vi "Multichannel Recording0.9EP.vi"() -> ()   [LabVIEW 2014]
uses:
  Consumer Data_ Consumer Event Com.ctl
  Data Producer States.ctl
  Enum State Typedef.ctl
  <vilib>/_DAQmxBase/Internals/DAQmxBase Read (Analog 2D DBL NChan NSamp).vi
  <vilib>/_DAQmxBase/Internals/DAQmxBase Create Channel (AI-Voltage-Basic).vi
  <vilib>/_DAQmxBase/Internals/DAQmxBase Timing (Sample Clock).vi
panel:
  out "Recording Progress (% )":dbl(slide) scale=0.0..1.0
  in  "Display Size":T1(ring)
  out "Data Producer State":T2=enum."Default"
  out "Data Consumer State":T3=enum."Default"
  in  "Open Button":bool
  in  "Tab Control":T4(tab)
  in  "Amplifier Channel 0":T5 {"Amplifier Model" items=["Select a Model", "AM 1700", "BMA 200"]}
  out "Channel 0 Graph":waveform(dbl)(graph)
  in  "User Data Channel 0":T6
  in  "Use Channel 0":bool caption="In Use?"
  out "Channel 1 Graph":waveform(dbl)(graph)
  in  "User Data Channel 1":T6
  in  "Amplifier Channel 1":T5 {"Amplifier Model" items=["Select a Model", "AM 1700", "BMA 200"]}
  in  "Use Channel 1":bool caption="In Use?"
  out "Channel 2 Graph":waveform(dbl)(graph)
  in  "User Data Channel 2":T6
  in  "Amplifier Channel 2":T5 {"Amplifier Model" items=["Select a Model", "AM 1700", "BMA 200"]}
  in  "Use Channel 2":bool caption="In Use?"
  out "Channel 3 Graph":waveform(dbl)(graph)
  in  "User Data Channel 3":T6
  in  "Amplifier Channel 3":T5 {"Amplifier Model" items=["Select a Model", "AM 1700", "BMA 200"]}
  in  "Use Channel 3":bool caption="In Use?"
  out "Overview Graph":waveform(dbl)[](graph)
  in  "Stop Preview":bool
  in  "OK Button":bool
  in  "Clear Display":bool
  in  "Preview Button":bool
  in  "Recording Time (s)":dbl
  in  "Sample Rate":i64=1000
  in  "Stop Button":bool
  out "Start Time hr/min":string
  out "Date mm/dd/yy":string
  in  "Exit Button":bool
  in  "Record Button":bool
  # "MSU EFISH Lab Multi-Channel Electronic Pulse Recorder v0.9E (Beta 6)"
  # "Setup"
  # "Must set sample rate before you press start"
  # "Preview"
  # "Recording"
  # "Blue for On\nOrange for Off"
  # "DC"
  # "AC"
  # "Blue for AC and Orange for DC"
  # "Blue for On\nOrange for Off"
  # "DC"
  # "AC"
  # "Blue for AC and Orange for DC"
  # "Blue for On\nOrange for Off"
  # "DC"
  # "AC"
  # "Blue for AC and Orange for DC"
  # "Blue for On\nOrange for Off"
  # "DC"
  # "AC"
  # "Blue for AC and Orange for DC"
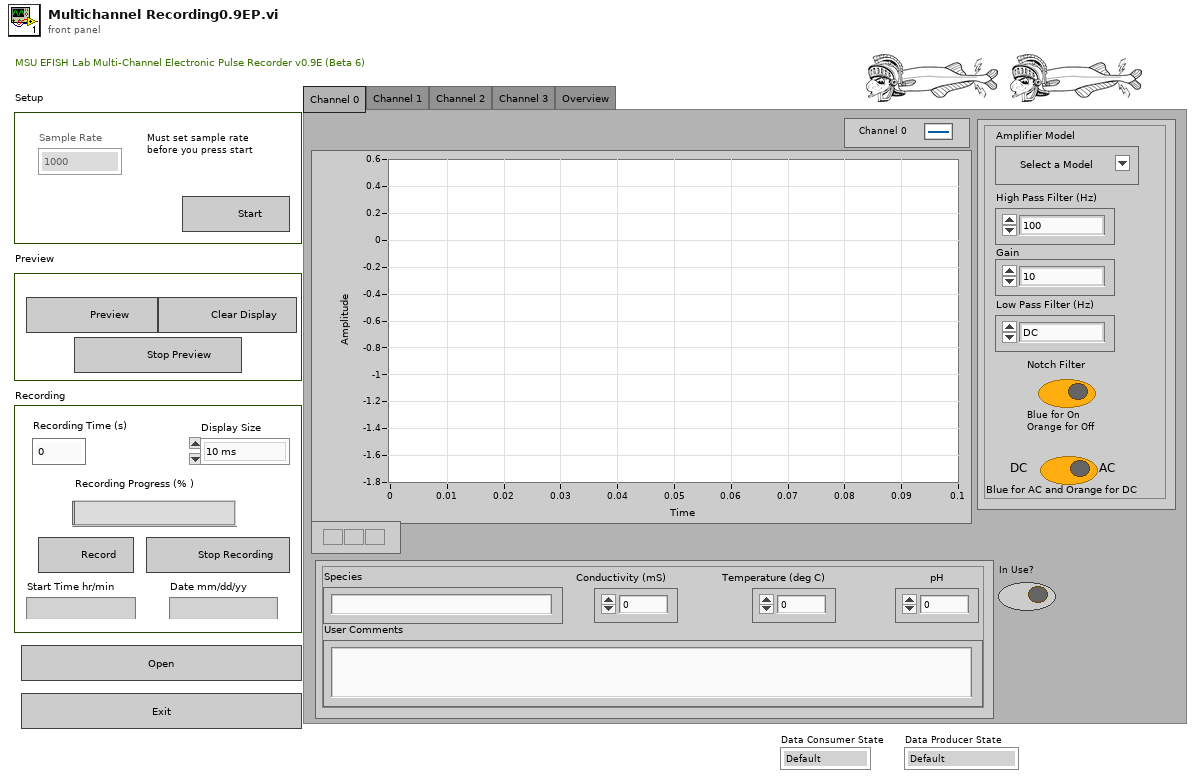
[diagram p1: front panel]
types:
  T1 = enum16{"10 ms", "100 ms", "1 Second", "10 sec", "30 sec"}
  T2 = typedef "Data Producer States.ctl" = enum16{"Read Data", "Set Sample Clock", "Default", "Exit", "Preview"}
  T3 = typedef "Consumer Data_ Consumer Event Com.ctl" = enum16{"Recording", "Create File", "Clear Memory", "Default", "End File", "Exit", "Set Sample Clock", "Preview"}
  T4 = enum32{"Channel 0", "Channel 1", "Channel 2", "Channel 3", "Overview"}
  T5 = cluster{"Low Pass Filter (Hz)":enum16{"DC", "0.1", "1", "3", "10", "30", "100", "300"}, "Gain ":enum16{"10", "20", "50", "100", "200", "500", "1000", "2k", "5k", "10k", "20k", "50k"}, "High Pass Filter (Hz)":enum16{"100", "500", "1000", "3000", "5000", "10,000", "20,000", "30,000", "50,000"}, "Notch Filter":bool, "Amplifier Model":u16, "AC/DC Switch":bool}
  T6 = cluster{"pH":dbl, "Conductivity (mS)":dbl, "Temperature (deg C)":dbl, "User Comments":string, "Species":string}
  T7 = enum8{"Enabled", "Disabled", "Disabled and Grayed Out"}
  T8 = cluster{"Overview Graph":refnum<vi>, "Channel 3 Graph":refnum<vi>, "Channel 2 Graph":refnum<vi>, "Channel 1 Graph":refnum<vi>, "Channel 0 Graph":refnum<vi>}
  T9 = typedef "Enum State Typedef.ctl" = enum16{"Default", "Open FIle", "Beginning State", "Set the Sample Clock", "Prepreview Handling", "Clear Display", "Preview Data", "Stop", "Exit", "Record", "Create File"}
  T10 = enum16{"Recording", "Create File", "Clear Memory", "Default"}
  T11 = cluster{"Refnum out":refnum<k34>, "Refnum out":refnum<k34>, "Refnum out":refnum<k34>, "Refnum out":refnum<k34>}
  T12 = cluster{"Use Channel 0":bool, "Use Channel 1":bool, "Use Channel 2":bool, "Use Channel 3":bool}
  T13 = cluster{"Waveform":waveform(dbl), "Waveform":waveform(dbl), "Waveform":waveform(dbl), "Waveform":waveform(dbl), waveform(dbl)[]}
  T14 = cluster{"tdms file out":refnum<k34>, "tdms file out":refnum<k34>, "tdms file out":refnum<k34>, "tdms file out":refnum<k34>}
  T15 = cluster{"User Data Channel 0":cluster{"pH":dbl, "Conductivity (mS)":dbl, "Temperature (deg C)":dbl, "User Comments":string, "Species":string}, "Amplifier Channel 0":cluster{"Low Pass Filter (Hz)":enum16{"DC", "0.1", "1", "3", "10", "30", "100", "300"}, "Gain ":enum16{"10", "20", "50", "100", "200", "500", "1000", "2k", "5k", "10k", "20k", "50k"}, "High Pass Filter (Hz)":enum16{"100", "500", "1000", "3000", "5000", "10,000", "20,000", "30,000", "50,000"}, "Notch Filter":bool, "Amplifier Model":u16, "AC/DC Switch":bool}, "User Data Channel 1":cluster{"pH":dbl, "Conductivity (mS)":dbl, "Temperature (deg C)":dbl, "User Comments":string, "Species":string}, "Amplifier Channel 1":cluster{"Low Pass Filter (Hz)":enum16{"DC", "0.1", "1", "3", "10", "30", "100", "300"}, "Gain ":enum16{"10", "20", "50", "100", "200", "500", "1000", "2k", "5k", "10k", "20k", "50k"}, "High Pass Filter (Hz)":enum16{"100", "500", "1000", "3000", "5000", "10,000", "20,000", "30,000", "50,000"}, "Notch Filter":bool, "Amplifier Model":u16, "AC/DC Switch":bool}, "User Data Channel 2":cluster{"pH":dbl, "Conductivity (mS)":dbl, "Temperature (deg C)":dbl, "User Comments":string, "Species":string}, "Amplifier Channel 2":cluster{"Low Pass Filter (Hz)":enum16{"DC", "0.1", "1", "3", "10", "30", "100", "300"}, "Gain ":enum16{"10", "20", "50", "100", "200", "500", "1000", "2k", "5k", "10k", "20k", "50k"}, "High Pass Filter (Hz)":enum16{"100", "500", "1000", "3000", "5000", "10,000", "20,000", "30,000", "50,000"}, "Notch Filter":bool, "Amplifier Model":u16, "AC/DC Switch":bool}, "User Data Channel 3":cluster{"pH":dbl, "Conductivity (mS)":dbl, "Temperature (deg C)":dbl, "User Comments":string, "Species":string}, "Amplifier Channel 3":cluster{"Low Pass Filter (Hz)":enum16{"DC", "0.1", "1", "3", "10", "30", "100", "300"}, "Gain ":enum16{"10", "20", "50", "100", "200", "500", "1000", "2k", "5k", "10k", "20k", "50k"}, "High Pass Filter (Hz)":enum16{"100", "500", "1000", "3000", "5000", "10,000", "20,000", "30,000", "50,000"}, "Notch Filter":bool, "Amplifier Model":u16, "AC/DC Switch":bool}}
  T16 = enum16{"Read Data", "Set Sample Clock", "Default", "Exit"}
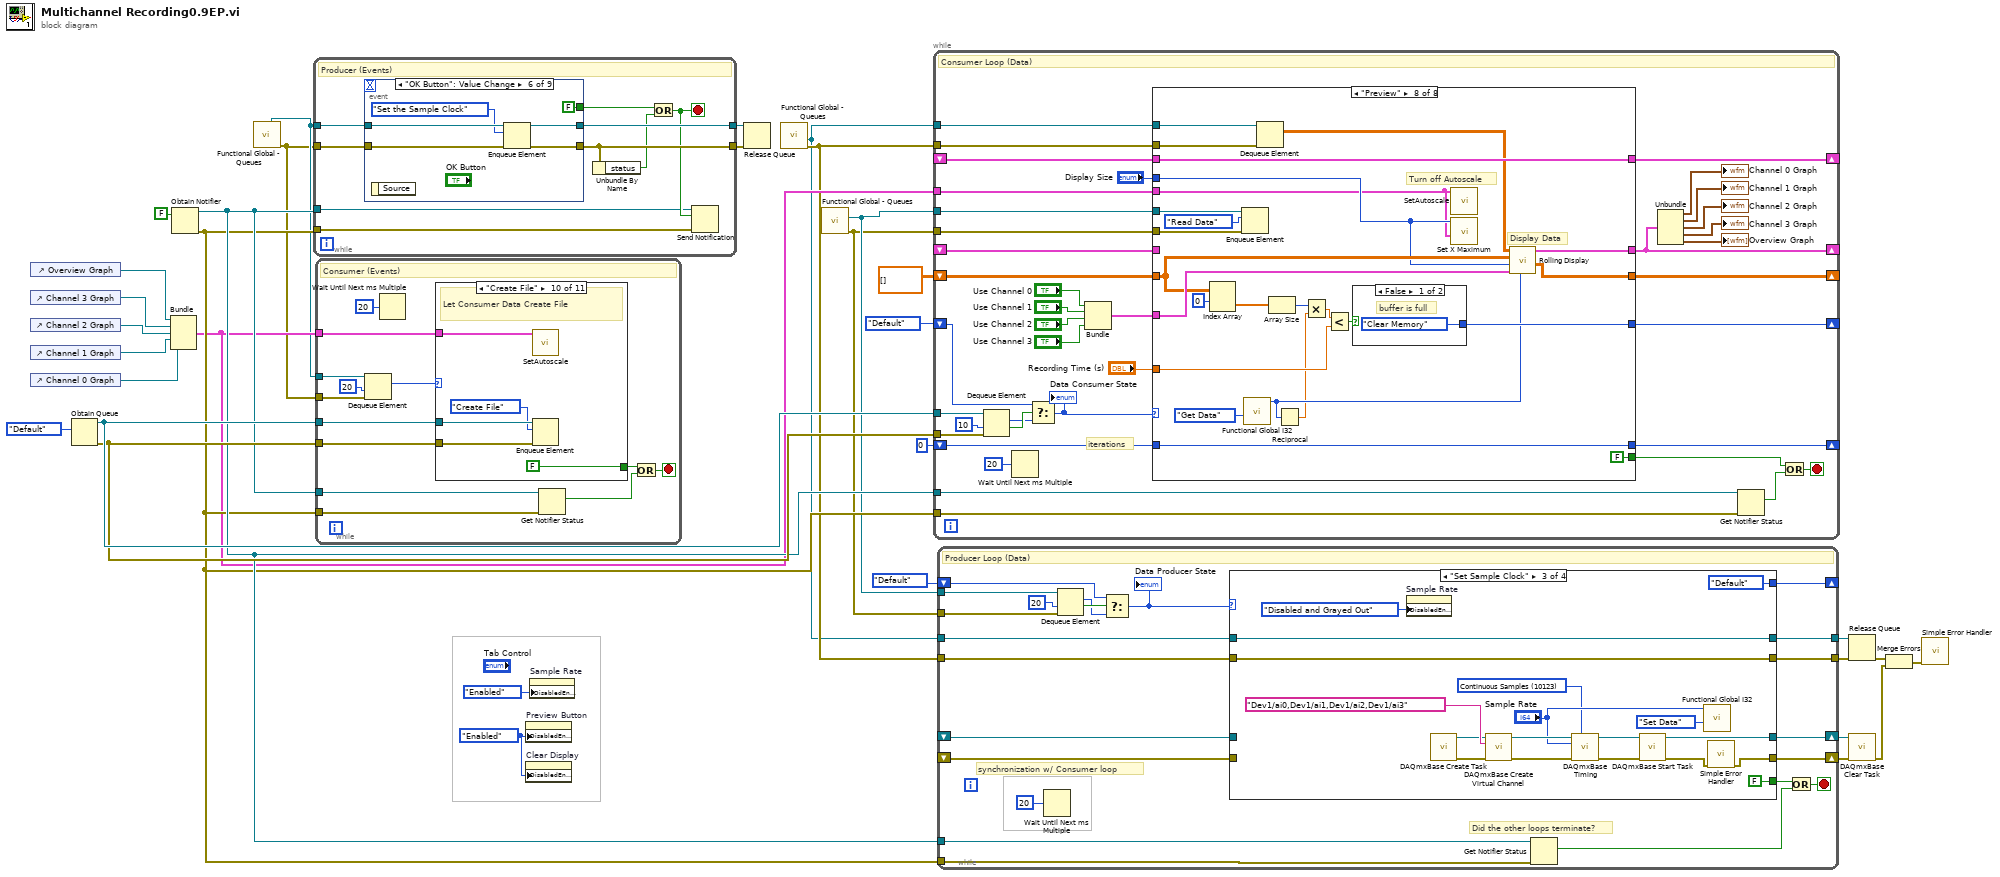
[diagram p0: block diagram]
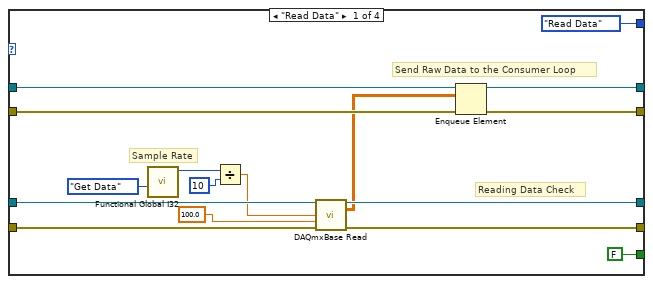
[diagram p2: hidden frame]
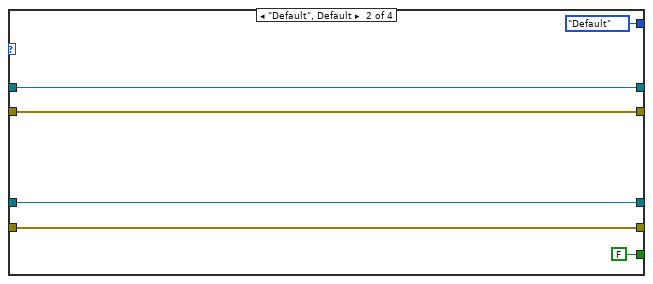
[diagram p3: hidden frame]
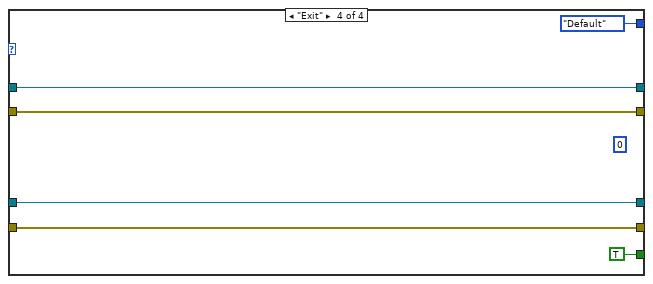
[diagram p4: hidden frame]
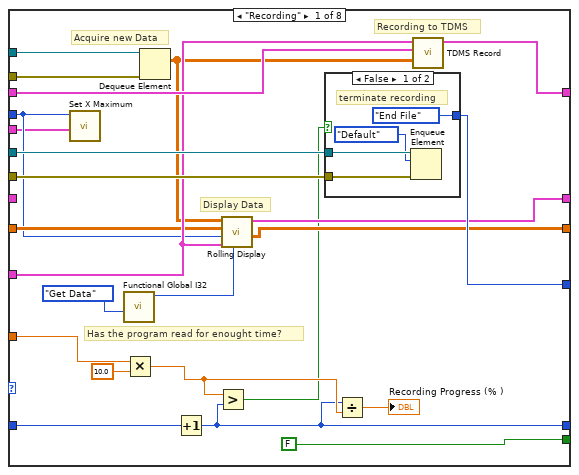
[diagram p5: hidden frame]
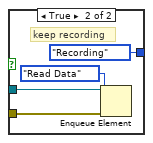
[diagram p6: hidden frame]
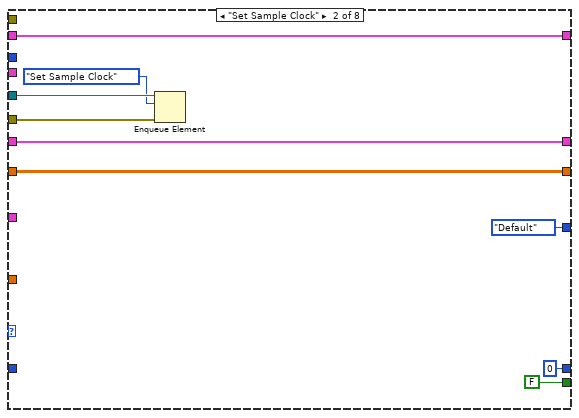
[diagram p7: hidden frame]
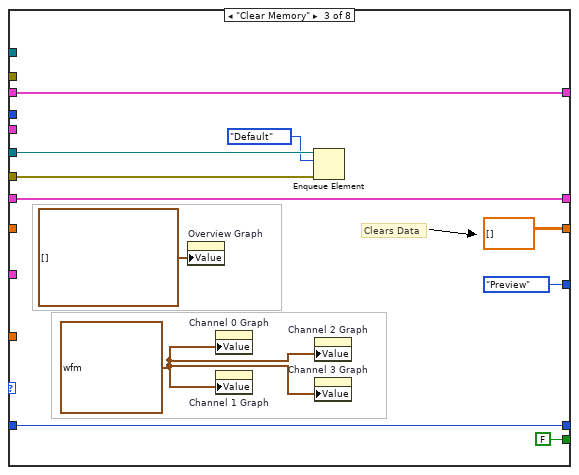
[diagram p8: hidden frame]
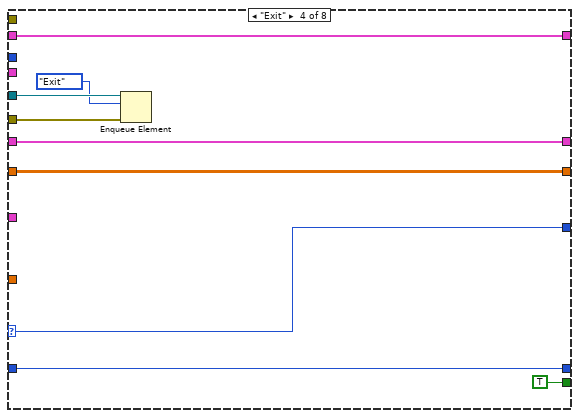
[diagram p9: hidden frame]
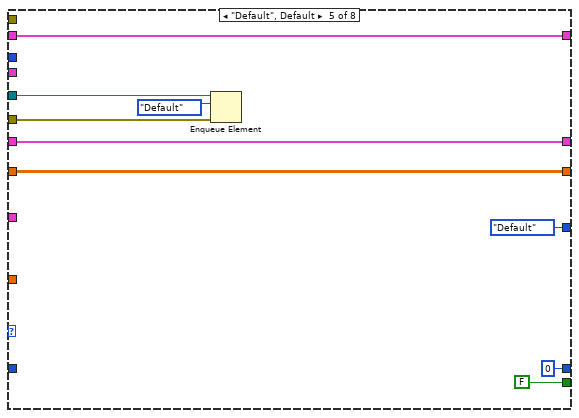
[diagram p10: hidden frame]
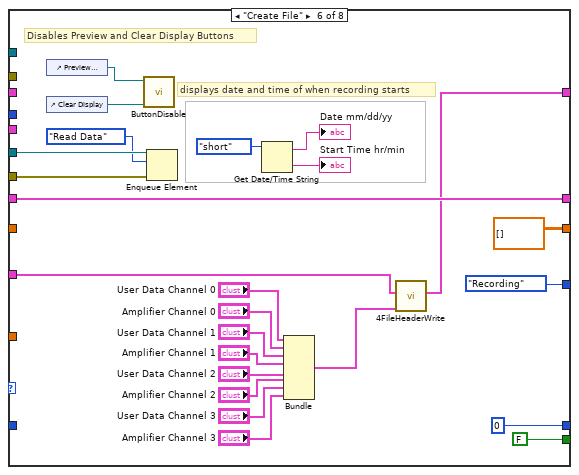
[diagram p11: hidden frame]
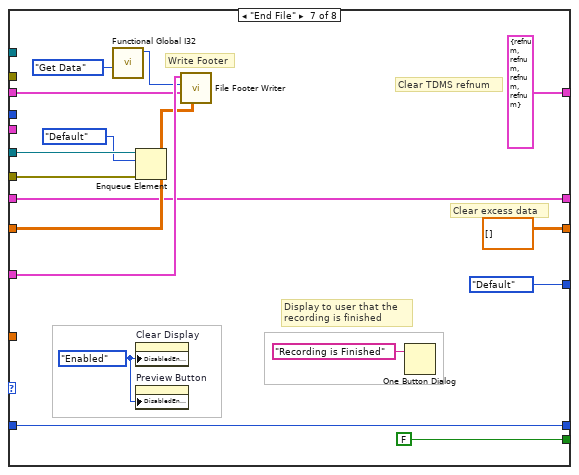
[diagram p12: hidden frame]
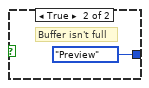
[diagram p13: hidden frame]
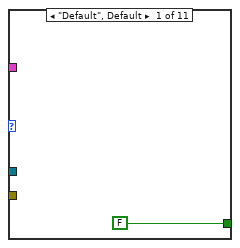
[diagram p14: hidden frame]
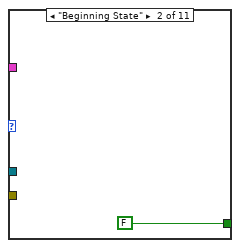
[diagram p15: hidden frame]
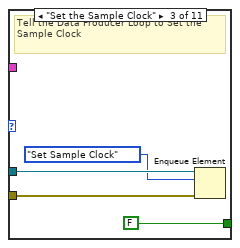
[diagram p16: hidden frame]
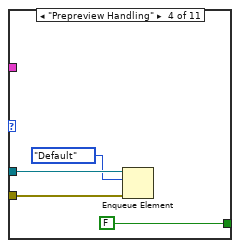
[diagram p17: hidden frame]
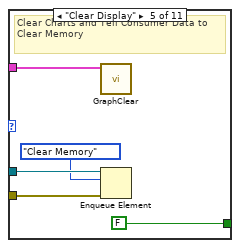
[diagram p18: hidden frame]
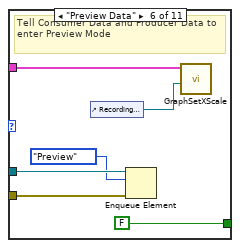
[diagram p19: hidden frame]
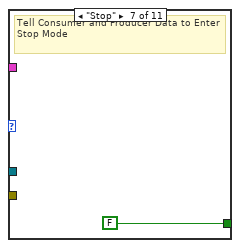
[diagram p20: hidden frame]
diagram:
  w13 = T7."Enabled" ("Disabled")
  n1 = control-ref of="Overview Graph"() -> (w12:refnum<vi>)
  n2 = control-ref of="Channel 3 Graph"() -> (w11:refnum<vi>)
  n3 = control-ref of="Channel 2 Graph"() -> (w10:refnum<vi>)
  n4 = control-ref of="Channel 1 Graph"() -> (w9:refnum<vi>)
  n5 = control-ref of="Channel 0 Graph"() -> (w8:refnum<vi>)
  n6 = Obtain Queue(element data type=Consumer_Data__Consumer_Event_Com."Default") -> (queue out=w29:refnum<queue>, error out=w28:errorcluster)  [unwired: 4 in, 1 out]
  n7 = Bundle("Overview Graph"=w12, "Channel 3 Graph"=w11, "Channel 2 Graph"=w10, "Channel 1 Graph"=w9, "Channel 0 Graph"=w8) -> (w7:T8)  [unwired: 1 in]
  n8 = Obtain Notifier(notification data type=FALSE) -> (notifier out=w15:refnum<notifier>, error out=w14:errorcluster)  [unwired: 3 in, 1 out]
  n9 = call "Functional Global - Queues.vi"() -> ("Error Out"=w1:errorcluster, "Producer Consumer Events Q"=w2:refnum<queue>)  [unwired: 7 in, 3 out]
  n10 = while {
    tunnel: w2 -> [w42]
    tunnel: w1 -> [w41]
    tunnel: [w40] -> w33
    tunnel: [w39] -> w32
    tunnel: w15 -> [w35]
    tunnel: w14 -> [w34]
    stop <- w36 stop-if-true
    # "Producer (Events)"
    n11 = event shown="[5] \"OK Button\": Value Change" {
      selector: _ -> [_ _ _ _ _ _ _ _ _]
      dyn-events: _ -> [_ _ _ _ _ _ _ _ _]
      timeout: _ -> [_ _ _ _ _ _ _ _ _]
      tunnel: [FALSE ("Exit Button") "Exit Button" FALSE ("Exit Button") FALSE ("Exit Button") FALSE ("Exit Button") FALSE ("Exit Button") FALSE ("Exit Button") FALSE ("Exit Button") FALSE ("Exit Button")] -> w38
      tunnel: w42 -> [w44 w50 w57 w63 w69 w75 w81 w87 w93]
      tunnel: w41 -> [w43 w49 w56 w62 w68 w74 w80 w86 w92]
      tunnel: [w44 w47 w53 w59 w65 w71 w77 w83 w89] -> w40
      tunnel: [w43 w46 w52 w58 w64 w70 w76 w82 w88] -> w39
      event Timeout {
        n12 = event-data() -> ()  [unwired: 1 in, 1 out]
      }
      event "Exit Button": Value Change {
        n13 = event-data() -> ()  [unwired: 1 in, 1 out]
        n14 = Enqueue Element(queue=w50, element=Enum_State_Typedef."Exit", error in (no error)=w49) -> (queue out=w47:refnum<queue>, error out=w46:errorcluster)  [unwired: 1 in, 1 out]
      }
      event "Preview Button": Value Change {
        n15 = event-data() -> ()  [unwired: 1 in, 1 out]
        n16 = Enqueue Element(queue=w57, element=Enum_State_Typedef."Preview Data", error in (no error)=w56) -> (queue out=w53:refnum<queue>, error out=w52:errorcluster)  [unwired: 1 in, 1 out]
      }
      event "Stop Preview": Value Change {
        n17 = event-data() -> ()  [unwired: 1 in, 1 out]
        n18 = Enqueue Element(queue=w63, element=Enum_State_Typedef."Prepreview Handling", error in (no error)=w62) -> (queue out=w59:refnum<queue>, error out=w58:errorcluster)  [unwired: 1 in, 1 out]
      }
      event "Open Button": Value Change {
        n19 = event-data() -> ()  [unwired: 1 in, 1 out]
        n20 = Enqueue Element(queue=w69, element=Enum_State_Typedef."Open FIle", error in (no error)=w68) -> (queue out=w65:refnum<queue>, error out=w64:errorcluster)  [unwired: 1 in, 1 out]
      }
      event "OK Button": Value Change {
        n21 = event-data() -> ()  [unwired: 1 in, 1 out]
        n22 = Enqueue Element(queue=w75, element=Enum_State_Typedef."Set the Sample Clock", error in (no error)=w74) -> (queue out=w71:refnum<queue>, error out=w70:errorcluster)  [unwired: 1 in, 1 out]
      }
      event "Stop Button": Value Change {
        n23 = event-data() -> ()  [unwired: 1 in, 1 out]
        n24 = Enqueue Element(queue=w81, element=Enum_State_Typedef."Stop", error in (no error)=w80) -> (queue out=w77:refnum<queue>, error out=w76:errorcluster)  [unwired: 1 in, 1 out]
      }
      event "Record Button": Value Change {
        n25 = event-data() -> ()  [unwired: 1 in, 1 out]
        n26 = Enqueue Element(queue=w87, element=Enum_State_Typedef."Create File", error in (no error)=w86) -> (queue out=w83:refnum<queue>, error out=w82:errorcluster)  [unwired: 1 in, 1 out]
      }
      event "Clear Display": Value Change {
        n27 = event-data() -> ()  [unwired: 1 in, 1 out]
        n28 = Enqueue Element(queue=w93, element=Enum_State_Typedef."Clear Display", error in (no error)=w92) -> (queue out=w89:refnum<queue>, error out=w88:errorcluster)  [unwired: 1 in, 1 out]
      }
    }
    n29 = Unbundle By Name(w39) -> ("status"=w37:bool)
    n30 = Or(x=w38, y=w37) -> (x .or. y?=w36:bool)
    n31 = Send Notification(notification=w36, notifier=w35, error in (no error)=w34) -> ()  [unwired: 2 out]
  }
  n32 = while {
    tunnel: w2 -> [w106]
    tunnel: w1 -> [w105]
    tunnel: w29 -> [w104]
    tunnel: w28 -> [w103]
    tunnel: w15 -> [w98]
    tunnel: w14 -> [w97]
    tunnel: w7 -> [w94]
    stop <- w96 stop-if-true
    # "Consumer (Events)"
    n33 = Dequeue Element(queue=w106, timeout in ms (-1)=20, error in (no error)=w105) -> (element=w101:T9)  [unwired: 3 out]
    n34 = Wait Until Next ms Multiple(millisecond multiple=u32 20) -> ()  [unwired: 1 out]
    n35 = case shown="\"Create File\"" w101 {
      tunnel: w104 -> [_ _ w111 w115 w120 w126 _ w132 _ w137 _]
      tunnel: w103 -> [_ _ w110 w114 w119 w125 _ w131 _ w136 _]
      tunnel: [FALSE FALSE FALSE FALSE FALSE FALSE FALSE TRUE FALSE FALSE FALSE] -> w102
      tunnel: w94 -> [_ _ _ _ w117 w122 _ _ _ w134 _]
      frame "Default", Default {
      }
      frame "Beginning State" {
      }
      frame "Set the Sample Clock" {
        # "Tell the Data Producer Loop to Set the Sample Clock"
        n36 = Enqueue Element(queue=w111, element=Consumer_Data__Consumer_Event_Com."Set Sample Clock", error in (no error)=w110) -> ()  [unwired: 1 in, 3 out]
      }
      frame "Prepreview Handling" {
        n37 = Enqueue Element(queue=w115, element=Consumer_Data__Consumer_Event_Com."Default", error in (no error)=w114) -> ()  [unwired: 1 in, 3 out]
      }
      frame "Clear Display" {
        # "Clear Charts and Tell Consumer Data to Clear Memory"
        n38 = call "GraphClear.vi"("Graph Reference Cluster"=w117) -> ()  [unwired: 11 in]
        n39 = Enqueue Element(queue=w120, element=Consumer_Data__Consumer_Event_Com."Clear Memory", error in (no error)=w119) -> ()  [unwired: 1 in, 3 out]
      }
      frame "Preview Data" {
        # "Tell Consumer Data and Producer Data to enter Preview Mode"
        n40 = control-ref of="Recording Time (s)"() -> (w123:refnum<vi>)
        n41 = Enqueue Element(queue=w126, element=Consumer_Data__Consumer_Event_Com."Preview", error in (no error)=w125) -> ()  [unwired: 1 in, 3 out]
        n42 = call "GraphSetXScale.vi"("Graph Reference Cluster"=w122, "Recording Time Reference"=w123) -> ()  [unwired: 9 in]
      }
      frame "Stop" {
        # "Tell Consumer and Producer Data to Enter Stop Mode"
      }
      frame "Exit" {
        # "Tell Producer and Consumer Data to end themselves then End the Program"
        n43 = Enqueue Element(queue=w132, element=Consumer_Data__Consumer_Event_Com."Exit", error in (no error)=w131) -> ()  [unwired: 1 in, 3 out]
      }
      frame "Record" {
        # "(I dont think that this case will exist)"
      }
      frame "Create File" {
        # "Let Consumer Data Create File"
        n44 = call "SetAutoscale.vi"("Cluster"=w134) -> ()  [unwired: 10 in]
        n45 = Enqueue Element(queue=w137, element=Consumer_Data__Consumer_Event_Com."Create File", error in (no error)=w136) -> ()  [unwired: 1 in, 3 out]
      }
      frame "Open FIle" {
        # "Tell the Data Consumer to Create the File"
        n46 = call "File Dialog"() -> ("selected path"=w139:path)  [unwired: 12 in, 3 out]
        n47 = call <vilib>:"TDMS - File Viewer.vi"("file path"=w139) -> ()  [unwired: 5 in, 2 out]
      }
    }
    n48 = Get Notifier Status(notifier=w98, error in (no error)=w97) -> (current notification=w95:bool)  [unwired: 4 out]
    n49 = Or(x=w102, y=w95) -> (x .or. y?=w96:bool)
  }
  n50 = property on="Preview Button" class="Bool (strict)"("DisabledEnum"=w13) -> ()  [unwired: 2 in, 2 out]
  n51 = property on="Clear Display" class="Bool"("DisabledEnum"=w13) -> ()  [unwired: 2 in, 2 out]
  n52 = property on="Sample Rate" class="DigNum (strict)"("DisabledEnum"=T7."Enabled" ("Disabled")) -> ()  [unwired: 2 in, 2 out]
  n53 = Release Queue(queue=w33, error in (no error)=w32) -> ()  [unwired: 1 in, 3 out]
  n54 = call "Functional Global - Queues.vi"() -> ("Error Out"=w6:errorcluster, "Data Q"=w5:refnum<queue>)  [unwired: 7 in, 3 out]
  n55 = call "Functional Global - Queues.vi"() -> ("Error Out"=w3:errorcluster, "Data Producer Control Q"=w4:refnum<queue>)  [unwired: 7 in, 3 out]
  n56 = while {
    tunnel: w5 -> [w172]
    tunnel: w6 -> [w171]
    tunnel: w29 -> [w179]
    tunnel: w28 -> [w178]
    shift-right: [w173] -> _
    shift-left: Consumer_Data__Consumer_Event_Com."Default" -> [w174]
    shift-right: [w167] -> _
    shift-left: dbl[][] [] -> [w170]
    shift-right: [w166] -> _
    shift-left: _ -> [w165]
    tunnel: w4 -> [w163]
    tunnel: w3 -> [w162]
    shift-right: [w158] -> _
    shift-left: 0 -> [w160]
    tunnel: w15 -> [w152]
    tunnel: w14 -> [w151]
    shift-right: [w144] -> _
    shift-left: _ -> [w143]
    tunnel: w7 -> [w141]
    stop <- w154 stop-if-true
    # "iterations"
    # "Consumer Loop (Data)"
    n57 = Dequeue Element(queue=w179, timeout in ms (-1)=10, error in (no error)=w178) -> (element=w176:T3, timed out?=w177:bool)  [unwired: 2 out]
    n58 = Wait Until Next ms Multiple(millisecond multiple=u32 20) -> ()  [unwired: 1 out]
    n59 = Select(t=w174, s=w177, f=w176) -> (s? t:f=w175:T3)
    "Data Consumer State" <- w175
    n60 = Bundle("Use Channel 0"="Use Channel 0", "Use Channel 1"="Use Channel 1", "Use Channel 2"="Use Channel 2", "Use Channel 3"="Use Channel 3") -> (w168:T12)  [unwired: 1 in]
    n61 = case shown="\"Preview\"" w175 {
      selector: w175 -> [_ _ _ w238 _ _ _ _]
      tunnel: [w196 Consumer_Data__Consumer_Event_Com."Default" Consumer_Data__Consumer_Event_Com."Preview" w238 T10."Default" Consumer_Data__Consumer_Event_Com."Recording" Consumer_Data__Consumer_Event_Com."Default" w308] -> w173
      tunnel: w172 -> [w202 _ _ _ _ _ _ w314]
      tunnel: w171 -> [w201 _ _ _ _ _ _ w313]
      tunnel: [FALSE FALSE FALSE TRUE FALSE FALSE FALSE FALSE] -> w153
      tunnel: w170 -> [w183 w217 _ w239 w247 _ w287 w296]
      tunnel: w168 -> [w191 _ _ _ _ w252 w289 w300]
      tunnel: [w189 w217 dbl[][] [] ("Output Decimated Data") w239 w247 dbl[][] [] ("Output Decimated Data") dbl[][] [] ("Output Data") w298] -> w167
      tunnel: [w200 w216 w228 w237 w246 w254 T11 {"Refnum out"=refnum, "Refnum out"=refnum, "Refnum out"=refnum, "Refnum out"=refnum} ("Output TDMS File Cluster") w301] -> w166
      tunnel: w165 -> [w193 w216 w228 w237 w246 _ w288 w301]
      tunnel: w163 -> [w195 w220 w227 w236 w244 w267 w282 w306]
      tunnel: w162 -> [w194 w219 w226 w235 w243 w266 w281 w305]
      tunnel: w160 -> [w199 _ w224 w233 _ _ w279 w303]
      tunnel: "Recording Time (s)" -> [w198 _ _ _ _ _ _ w297]
      tunnel: [w186 0 w224 w233 0 0 w279 w303] -> w158
      tunnel: [w190 w212 w223 w232 w241 w263 w277 w299] -> w144
      tunnel: w143 -> [_ w212 w223 w232 w241 w263 w277 _]
      tunnel: "Display Size" -> [w182 _ _ _ _ _ _ w293]
      tunnel: w141 -> [w180 _ _ _ _ _ _ w290]
      frame "Recording" {
        # "Acquire new Data"
        # "Has the program read for enought time?"
        # "Display Data"
        # "Recording to TDMS"
        n62 = call "Set X Maximum.vi"("Cluster"=w180, "Display Size"=w182) -> ()  [unwired: 10 in]
        n63 = call "Functional Global I32.vi"("Enum"=enum16{"Set Data", "Get Data"}."Get Data") -> ("Integer"=w181:i32)  [unwired: 10 in]
        n64 = Multiply(x=w198, y=10.0) -> (x*y=w187:dbl)
        n65 = Dequeue Element(queue=w202, error in (no error)=w201) -> (element=w184:dbl[][])  [unwired: 1 in, 3 out]
        n66 = Increment(x=w199) -> (x+1=w186:i32)
        n67 = Greater?(x=w187, y=w186) -> (0:w185:bool)
        n68 = call "Rolling Display.vi"("Sample Rate"=w181, "Channels in Use"=w191, "Display Size"=w182, "Old Data"=w183, "Input Data"=w184) -> ("Output Array Values"=w189:dbl[][], "Output Waveform Cluster"=w190:T13)  [unwired: 5 in]
        n69 = case shown="False" w185 {
          tunnel: [Consumer_Data__Consumer_Event_Com."End File" Consumer_Data__Consumer_Event_Com."Recording"] -> w196
          tunnel: w195 -> [w206 w210]
          tunnel: w194 -> [w205 w209]
          frame False {
            # "terminate recording"
            n70 = Enqueue Element(queue=w206, element=Data_Producer_States."Default", error in (no error)=w205) -> ()  [unwired: 1 in, 3 out]
          }
          frame True {
            # "keep recording"
            n71 = Enqueue Element(queue=w210, element=Data_Producer_States."Read Data", error in (no error)=w209) -> ()  [unwired: 1 in, 3 out]
          }
        }
        n72 = Divide(x=w186, y=w187) -> (x/y=→"Recording Progress (% )":dbl)
        n73 = call "TDMS Record.vi"("Data"=w184, "Input TDMS File Cluster"=w193, "In Use Cluster"=w191) -> ("Output TDMS File Cluster"=w200:T14)  [unwired: 8 in]
      }
      frame "Set Sample Clock" {
        n74 = Enqueue Element(queue=w220, element=Data_Producer_States."Set Sample Clock", error in (no error)=w219) -> ()  [unwired: 1 in, 3 out]
      }
      frame "Clear Memory" {
        w222 = waveform(dbl) {"t0"=timestamp(0 s since 1904-01-01), "dt"=1.0, "Y"=[]} ("Channel 0 Graph")
        # "Clears Data"
        n75 = property on="Overview Graph" class="WFGraph (strict)"("Value"=waveform(dbl)[] [] ("Overview Graph")) -> ()  [unwired: 2 in, 2 out]
        n76 = property on="Channel 0 Graph" class="WFGraph (strict)"("Value"=w222) -> ()  [unwired: 2 in, 2 out]
        n77 = property on="Channel 1 Graph" class="WFGraph (strict)"("Value"=w222) -> ()  [unwired: 2 in, 2 out]
        n78 = Enqueue Element(queue=w227, element=Data_Producer_States."Default", error in (no error)=w226) -> ()  [unwired: 1 in, 3 out]
        n79 = property on="Channel 2 Graph" class="WFGraph (strict)"("Value"=w222) -> ()  [unwired: 2 in, 2 out]
        n80 = property on="Channel 3 Graph" class="WFGraph (strict)"("Value"=w222) -> ()  [unwired: 2 in, 2 out]
      }
      frame "Exit" {
        n81 = Enqueue Element(queue=w236, element=Data_Producer_States."Exit", error in (no error)=w235) -> ()  [unwired: 1 in, 3 out]
      }
      frame "Default", Default {
        n82 = Enqueue Element(queue=w244, element=Data_Producer_States."Default", error in (no error)=w243) -> ()  [unwired: 1 in, 3 out]
      }
      frame "Create File" {
        # "displays date and time of when recording starts"
        # "Disables Preview and Clear Display Buttons"
        n83 = control-ref of="Preview Button"() -> (w250:refnum<vi>)
        n84 = control-ref of="Clear Display"() -> (w251:refnum<vi>)
        n85 = call "ButtonDisable.vi"("Clear Display Button Reference"=w251, "Preview Button Reference"=w250) -> ()  [unwired: 10 in]
        n86 = Enqueue Element(queue=w267, element=Data_Producer_States."Read Data", error in (no error)=w266) -> ()  [unwired: 1 in, 3 out]
        n87 = Get Date/Time String(date format (0)=enum16{"short", "long", "abbreviated"}."short") -> (date string=→"Date mm/dd/yy":string, time string=→"Start Time hr/min":string)  [unwired: 2 in]
        n88 = Bundle("User Data Channel 0"="User Data Channel 0", "Amplifier Channel 0"="Amplifier Channel 0", "User Data Channel 1"="User Data Channel 1", "Amplifier Channel 1"="Amplifier Channel 1", "User Data Channel 2"="User Data Channel 2", "Amplifier Channel 2"="Amplifier Channel 2", "User Data Channel 3"="User Data Channel 3", "Amplifier Channel 3"="Amplifier Channel 3") -> (w253:T15)  [unwired: 1 in]
        n89 = call "4FileHeaderWrite.vi"("MetaData Cluster"=w253, "In Use Cluster"=w252) -> ("Cluster out"=w254:T11)  [unwired: 9 in]
      }
      frame "End File" {
        w276 = T7."Enabled" ("Disabled")
        # "Write Footer"
        # "Clear TDMS refnum"
        # "Clear excess data"
        # "Display to user that the \nrecording is finished"
        n90 = call "Functional Global I32.vi"("Enum"=enum16{"Set Data", "Get Data"}."Get Data") -> ("Integer"=w274:i32)  [unwired: 10 in]
        n91 = Enqueue Element(queue=w282, element=Data_Producer_States."Default", error in (no error)=w281) -> ()  [unwired: 1 in, 3 out]
        n92 = property on="Clear Display" class="Bool"("DisabledEnum"=w276) -> ()  [unwired: 2 in, 2 out]
        n93 = property on="Preview Button" class="Bool (strict)"("DisabledEnum"=w276) -> ()  [unwired: 2 in, 2 out]
        n94 = call "File Footer Writer.vi"("Old Data"=w287, "TDMS File Cluster"=w288, "Sample Rate"=w274, "In Use Cluster"=w289) -> ()  [unwired: 8 in]
        n95 = One Button Dialog(message="Recording is Finished") -> ()  [unwired: 1 in, 1 out]
      }
      frame "Preview" {
        # "Display Data"
        # "Turn off Autoscale"
        n96 = Index Array(array=w296, index (row)=0) -> (element=w311:dbl[])  [unwired: 1 in]
        n97 = Enqueue Element(queue=w306, element=Data_Producer_States."Read Data", error in (no error)=w305) -> ()  [unwired: 1 in, 3 out]
        n98 = call "Functional Global I32.vi"("Enum"=enum16{"Set Data", "Get Data"}."Get Data") -> ("Integer"=w294:i32)  [unwired: 10 in]
        n99 = Dequeue Element(queue=w314, error in (no error)=w313) -> (element=w295:dbl[][])  [unwired: 1 in, 3 out]
        n100 = Array Size(array=w311) -> (size(s)=w291:i32)
        n101 = Reciprocal(x=w294) -> (1/x=w292:dbl)
        n102 = Multiply(x=w291, y=w292) -> (x*y=w310:dbl)
        n103 = Less?(x=w310, y=w297) -> (x < y?=w309:bool)
        n104 = case shown="False" w309 {
          tunnel: [Consumer_Data__Consumer_Event_Com."Clear Memory" Consumer_Data__Consumer_Event_Com."Preview"] -> w308
          frame False {
            # "buffer is full"
          }
          frame True {
            # "Buffer isn't full"
          }
        }
        n105 = call "SetAutoscale.vi"("Cluster"=w290) -> ()  [unwired: 10 in]
        n106 = call "Set X Maximum.vi"("Cluster"=w290, "Display Size"=w293) -> ()  [unwired: 10 in]
        n107 = call "Rolling Display.vi"("Sample Rate"=w294, "Channels in Use"=w300, "Display Size"=w293, "Old Data"=w296, "Input Data"=w295) -> ("Output Array Values"=w298:dbl[][], "Output Waveform Cluster"=w299:T13)  [unwired: 5 in]
      }
    }
    n108 = Unbundle(w144) -> ("Waveform"=→"Channel 0 Graph":waveform(dbl), "Waveform"=→"Channel 1 Graph":waveform(dbl), "Waveform"=→"Channel 2 Graph":waveform(dbl), "Waveform"=→"Channel 3 Graph":waveform(dbl), →"Overview Graph":waveform(dbl)[])
    n109 = Get Notifier Status(notifier=w152, error in (no error)=w151) -> (current notification=w150:bool)  [unwired: 4 out]
    n110 = Or(x=w153, y=w150) -> (x .or. y?=w154:bool)
  }
  n111 = while {
    tunnel: w5 -> [w338]
    tunnel: w6 -> [w335]
    tunnel: [w337] -> w31
    tunnel: [w336] -> w30
    shift-right: [w323] -> _
    shift-left: Data_Producer_States."Default" -> [w318]
    shift-right: [w334] -> w26
    shift-left: _ -> [w332]
    shift-right: [w333] -> w25
    shift-left: _ -> [w331]
    tunnel: w4 -> [w328]
    tunnel: w3 -> [w327]
    tunnel: w15 -> [w320]
    tunnel: w14 -> [w319]
    stop <- w322 stop-if-true
    # "synchronization w/ Consumer loop"
    # "Did the other loops terminate?"
    # "Producer Loop (Data)"
    n112 = Wait Until Next ms Multiple(millisecond multiple=u32 20) -> ()  [unwired: 1 out]
    n113 = Dequeue Element(queue=w328, timeout in ms (-1)=20, error in (no error)=w327) -> (element=w317:T2, timed out?=w326:bool)  [unwired: 2 out]
    n114 = Select(t=w318, s=w326, f=w317) -> (s? t:f=w325:T2)
    "Data Producer State" <- w325
    n115 = case shown="\"Set Sample Clock\"" w325 {
      tunnel: w338 -> [w350 w360 w370 w380]
      tunnel: [w348 w360 w370 w380] -> w337
      tunnel: [w347 w359 w369 w381] -> w336
      tunnel: w335 -> [w349 w359 w369 w381]
      tunnel: [w352 w358 w371 w382] -> w334
      tunnel: [w351 w357 w361 w383] -> w333
      tunnel: w332 -> [w354 w358 _ w382]
      tunnel: w331 -> [w353 w357 _ w383]
      tunnel: [FALSE FALSE FALSE TRUE] -> w329
      tunnel: [Data_Producer_States."Read Data" Data_Producer_States."Default" T16."Default" Data_Producer_States."Default"] -> w323
      frame "Read Data" {
        # "Send Raw Data to the Consumer Loop"
        # "Reading Data Check"
        # "Sample Rate"
        n116 = call "Functional Global I32.vi"("Enum"=enum16{"Set Data", "Get Data"}."Get Data") -> ("Integer"=w341:i32)  [unwired: 10 in]
        n117 = Divide(x=w341, y=10) -> (x/y=w340:dbl)
        n118 = call-poly <vilib>:"DAQmxBase Read.vi"("task/channels in"=w354, "number of samples per channel"=w340, "timeout"=100.0, "error in"=w353) -> ("task out"=w352:refnum<k21>, "data"=w339:dbl[][], "error out"=w351:errorcluster)  [unwired: 9 in]
        n119 = Enqueue Element(queue=w350, element=w339, error in (no error)=w349) -> (queue out=w348:refnum<queue>, error out=w347:errorcluster)  [unwired: 1 in, 1 out]
      }
      frame "Default", Default {
      }
      frame "Set Sample Clock" {
        w363 = 10123 items=["Finite Samples"=10178, "Continuous Samples"=10123, "Hardware Timed Single Point"=12522] ("sample mode")
        n120 = property on="Sample Rate" class="DigNum (strict)"("DisabledEnum"=T7."Disabled and Grayed Out" ("Disabled")) -> ()  [unwired: 2 in, 2 out]
        n121 = call <vilib>:"DAQmxBase Create Task.vi"() -> ("task out"=w377:refnum<k21>, "error out"=w376:errorcluster)  [unwired: 14 in]
        n122 = call-poly <vilib>:"DAQmxBase Create Virtual Channel.vi"("task in"=w377, "physical channels"=tag "Dev1/ai0,Dev1/ai1,Dev1/ai2,Dev1/ai3", "error in"=w376) -> ("task out"=w374:refnum<k21>, "error out"=w375:errorcluster)  [unwired: 11 in]
        n123 = call-poly <vilib>:"DAQmxBase Timing.vi"("task/channels in"=w374, "sample mode"=w363, "rate"="Sample Rate", "error in"=w375) -> ("task out"=w373:refnum<k21>, "error out"=w372:errorcluster)  [unwired: 10 in]
        n124 = call <vilib>:"DAQmxBase Start Task.vi"("task/channels in"=w373, "error in"=w372) -> ("task out"=w371:refnum<k21>, "error out"=w362:errorcluster)  [unwired: 12 in]
        n125 = call "Functional Global I32.vi"("Enum"=enum16{"Set Data", "Get Data"}."Set Data", "Integer In"="Sample Rate") -> ()  [unwired: 9 in, 1 out]
        n126 = call <vilib>:"Simple Error Handler.vi"("error in (no error)"=w362) -> ("error out"=w361:errorcluster)  [unwired: 4 in, 4 out]
      }
      frame "Exit" {
        (unwired) 0
      }
    }
    n127 = Get Notifier Status(notifier=w320, error in (no error)=w319) -> (current notification=w321:bool)  [unwired: 4 out]
    n128 = Or(x=w329, y=w321) -> (x .or. y?=w322:bool)
  }
  n129 = Release Queue(queue=w31, error in (no error)=w30) -> (error out=w24:errorcluster)  [unwired: 1 in, 2 out]
  n130 = call <vilib>:"DAQmxBase Clear Task.vi"("task in"=w26, "error in"=w25) -> ("error out"=w23:errorcluster)  [unwired: 13 in]
  n131 = Merge Errors(w24, w23) -> (w22:errorcluster)
  n132 = call <vilib>:"Simple Error Handler.vi"("error in (no error)"=w22) -> ()  [unwired: 4 in, 5 out]
